vi "Part 1.vi"(11 "Input":string) -> (2 "Incomplete Stacks":cluster{"Stack":string[]}[](array[cluster]), 3 "Output":i64)   [LabVIEW 2021]
panel:
  out "Corrupt Characters":string[](array[string])
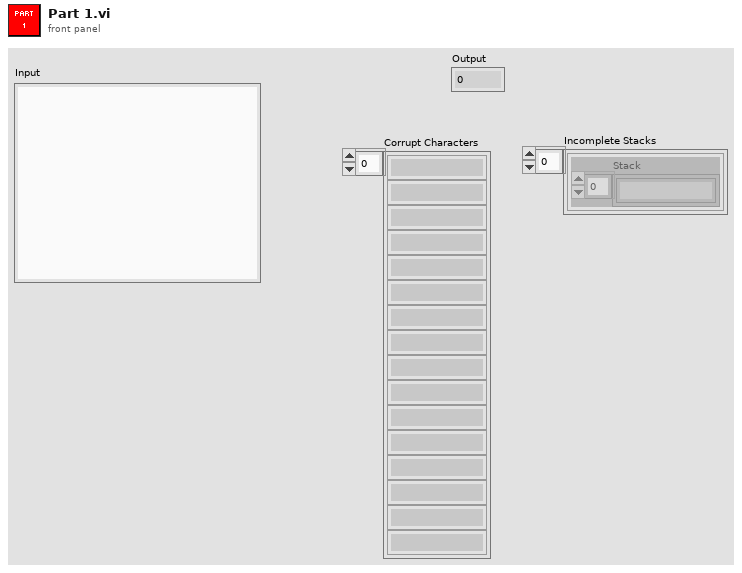
[diagram p1: front panel]
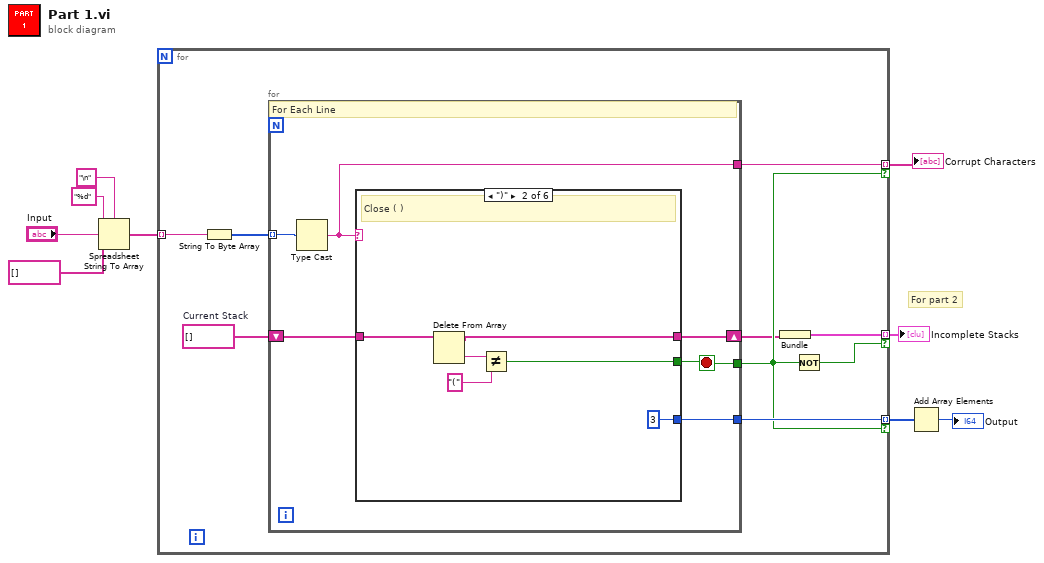
[diagram p0: block diagram]
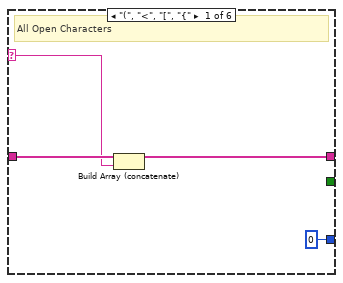
[diagram p2: hidden frame]
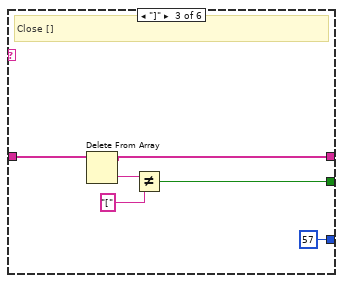
[diagram p3: hidden frame]
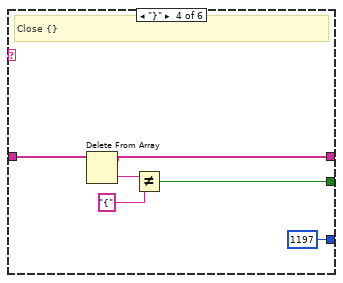
[diagram p4: hidden frame]
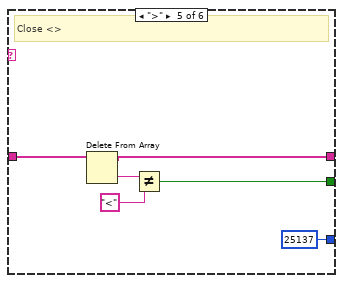
[diagram p5: hidden frame]
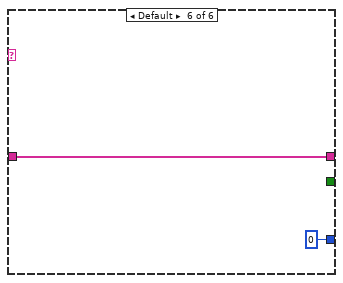
[diagram p6: hidden frame]
diagram:
  # "For part 2"
  n1 = Spreadsheet String To Array(delimiter (Tab)="\n", format string="%d", spreadsheet string="Input", array type (2D Dbl)=string[] []) -> (array=w5:string[])
  n2 = for {
    tunnel: w5 -> [w16] mode=indexing
    tunnel: [w15] -> w4 mode=indexing if=w13
    tunnel: [w14] -> w3 mode=indexing if=w13
    tunnel: [w11] -> w1 mode=indexing if=w10
    w17 = string[] []  # Current Stack
    n3 = String To Byte Array(string=w16) -> (unsigned byte array=w18:u8[])
    n4 = for {
      tunnel: w18 -> [w24] mode=indexing
      shift-right: [w22] -> w12
      shift-left: w17 -> [w23]
      tunnel: [w21] -> w15
      tunnel: [w20] -> w13
      tunnel: [w19] -> w14
      stop <- w20 stop-if-true
      # "For Each Line"
      n5 = Type Cast(x=w24) -> (*(type *) &x=w21:string)  [unwired: 1 in]
      n6 = case shown="\")\"" w21 {
        selector: w21 -> [w27 _ _ _ _ _]
        tunnel: w23 -> [w28 w34 w40 w46 w52 w54]
        tunnel: [w26 w33 w39 w45 w51 w54] -> w22
        tunnel: [_ w30 w36 w42 w48 _] -> w20
        tunnel: [0 3 57 1197 25137 0] -> w19
        frame "(", "<", "[", "{" {
          # "All Open Characters"
          n7 = Build Array (concatenate)(w28, w27) -> (w26:string[])
        }
        frame ")" {
          # "Close ( )"
          n8 = Delete From Array(array=w34) -> (deleted portion=w32:string, array with subset deleted=w33:string[])  [unwired: 2 in]
          n9 = Not Equal?(x=w32, y="(") -> (x != y?=w30:bool)
        }
        frame "]" {
          # "Close []"
          n10 = Delete From Array(array=w40) -> (deleted portion=w38:string, array with subset deleted=w39:string[])  [unwired: 2 in]
          n11 = Not Equal?(x=w38, y="[") -> (x != y?=w36:bool)
        }
        frame "}" {
          # "Close {}"
          n12 = Delete From Array(array=w46) -> (deleted portion=w44:string, array with subset deleted=w45:string[])  [unwired: 2 in]
          n13 = Not Equal?(x=w44, y="{") -> (x != y?=w42:bool)
        }
        frame ">" {
          # "Close <>"
          n14 = Delete From Array(array=w52) -> (deleted portion=w50:string, array with subset deleted=w51:string[])  [unwired: 2 in]
          n15 = Not Equal?(x=w50, y="<") -> (x != y?=w48:bool)
        }
        frame Default {
        }
      }
    }
    n16 = Bundle("Current Stack"=w12) -> (w11:cluster{"Current Stack":string[]})  [unwired: 1 in]
    n17 = Not(x=w13) -> (.not. x?=w10:bool)
  }
  "Corrupt Characters" <- w4
  "Incomplete Stacks" <- w1
  n18 = Add Array Elements(numeric array=w3) -> (sum=→"Output":i32)
